vi "Set RX SW.vi"(0 "NMR in":refnum<class "NMR.lvclass">, 5 "On/Off":bool, 11 "error in (no error)":errorcluster) -> (4 "NMR out":refnum<class "NMR.lvclass">, 10 "String as ASCII":string, 15 "error out":errorcluster)   [LabVIEW 2011, in "NMR.lvclass"]
uses:
  NMR.lvclass
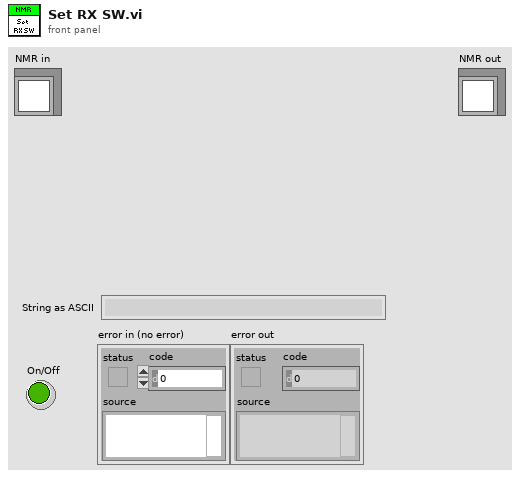
[diagram p1: front panel]
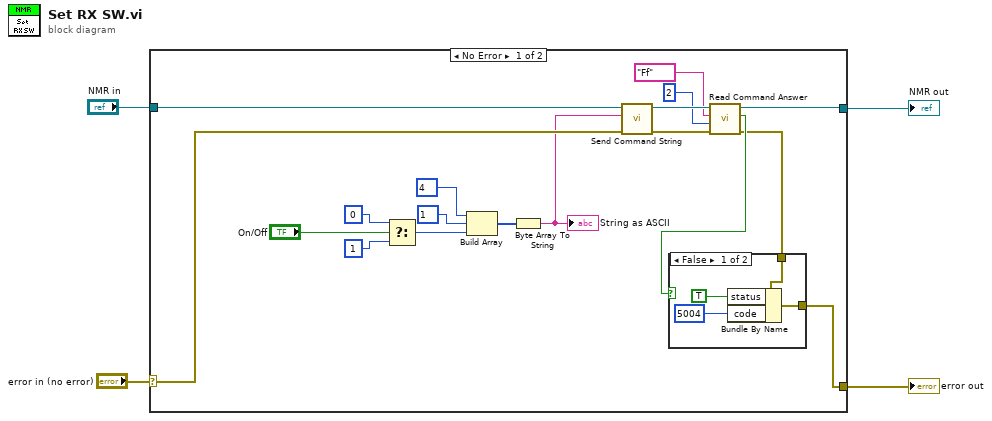
[diagram p0: block diagram]
diagram:
  n1 = case shown="No Error" "error in (no error)" {
    selector: "error in (no error)" -> [w19 w29]
    tunnel: [w10 w29] -> w3
    tunnel: [w20 w28] -> w1
    tunnel: "NMR in" -> [w22 w28]
    frame No Error {
      n2 = Select(t=u8 0, s="On/Off", f=u8 1) -> (s? t:f=w5:u8)
      n3 = Build Array(u32 4 ("element"), u32 1 ("element"), w5) -> (w17:u32[])
      n4 = Byte Array To String(unsigned byte array=w17) -> (string=w15:string)
      "String as ASCII" <- w15
      n5 = call-dynamic "Send Command String.vi"("error in (no error)"=w19, "Command String"=w15, "NMR in"=w22) -> ("error out"=w18:errorcluster, "NMR out"=w21:refnum<class "NMR.lvclass">)  [unwired: 7 in]
      n6 = call-dynamic "Read Command Answer.vi"("error in (no error)"=w18, "bytes to read"=u32 2 ("Number bytes Read"), "String Seached"="Ff" ("search char"), "NMR in"=w21) -> ("error out"=w11:errorcluster, "Expected Answer?"=w12:bool, "NMR out"=w20:refnum<class "NMR.lvclass">)  [unwired: 5 in]
      n7 = case shown="False" w12 {
        tunnel: w11 -> [w24 w27]
        tunnel: [w23 w27] -> w10
        frame False {
          n8 = Bundle By Name(cluster=w24, "status"=TRUE, "code"=5004) -> (w23:errorcluster)
        }
        frame True {
        }
      }
    }
    frame Error {
    }
  }
  "error out" <- w3
  "NMR out" <- w1
